vi "Initialize.vi"(6 "optional":variant, 8 "error in":errorcluster, 11 "FPGADMAChannelData in":refnum<class "FPGADMAChannelData.lvclass">) -> (0 "error out":errorcluster, 3 "Node*":refnum<data-value>)   [LabVIEW 2013, in "FPGADMAChannelData.lvclass"]
uses:
  FPGADMAChannelData.lvclass
  xCE/xceNode/xceNode.lvclass
  Categories/Categories.lvclass
  DMA_Read/DMA_Read.lvclass
  DMA_Write/DMA_Write.lvclass
  Category/Category.lvclass
  xCE/xceRootNode/xceRootNode.lvclass
  xCE/xceDataNode/xceDataNode.lvclass
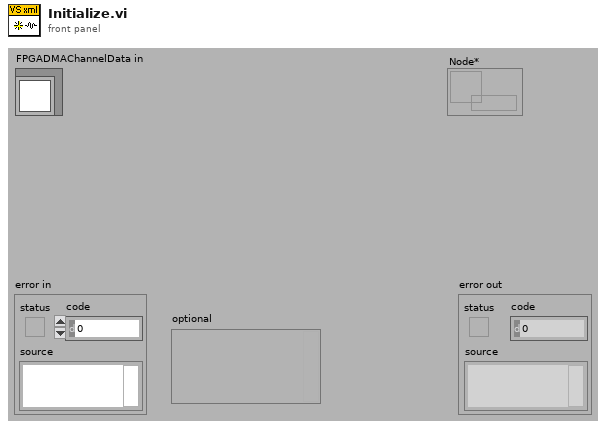
[diagram p1: front panel]
types:
  T1 = cluster{"className":string, "classAlias":string}[]
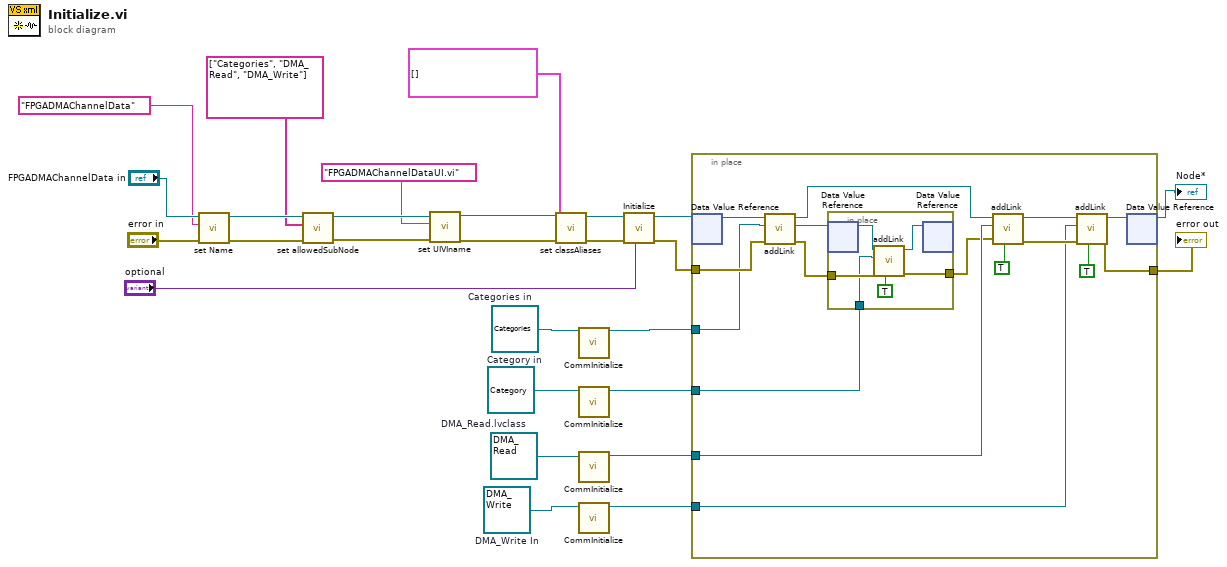
[diagram p0: block diagram]
diagram:
  w7 = refnum<class "Category.lvclass"> refnum  # Category in
  w13 = refnum<class "DMA_Write.lvclass"> refnum  # DMA_Write In
  w14 = refnum<class "DMA_Read.lvclass"> refnum  # DMA_Read.lvclass
  w15 = refnum<class "Categories.lvclass"> refnum  # Categories in
  n1 = call "set Name.vi"("error in (no error)"="error in", "Name"="FPGADMAChannelData", "xceDataNode in"="FPGADMAChannelData in") -> ("error out"=w22:errorcluster, "xceDataNode out"=w23:refnum<class "FPGADMAChannelData.lvclass">)  [unwired: 7 in]
  n2 = call "set allowedSubNode.vi"("error in (no error)"=w22, "Allowed subNode[]"=string[] ["Categories", "DMA_Read", "DMA_Write"], "xceDataNode in"=w23) -> ("error out"=w19:errorcluster, "xceDataNode out"=w20:refnum<class "FPGADMAChannelData.lvclass">)  [unwired: 7 in]
  n3 = call "set UIVIname.vi"("error in (no error)"=w19, "UI VI name"="FPGADMAChannelDataUI.vi", "xceDataNode in"=w20) -> ("error out"=w2:errorcluster, "xceDataNode out"=w5:refnum<class "FPGADMAChannelData.lvclass">)  [unwired: 7 in]
  n4 = call "set classAliases.vi"("error in (no error)"=w2, "classAliases"=T1 [], "xceRootNode in"=w5) -> ("error out"=w3:errorcluster, "xceRootNode out"=w4:refnum<class "FPGADMAChannelData.lvclass">)  [unwired: 7 in]
  n5 = call "CommInitialize.vi"("Categories in"=w15) -> ("Node*"=w12:refnum<data-value>)  [unwired: 9 in, 1 out]
  n6 = call "CommInitialize.vi"("Category in"=w7) -> ("Node*"=w6:refnum<data-value>)  [unwired: 9 in, 1 out]
  n7 = call "CommInitialize.vi"("DMA_Read.lvclass"=w14) -> ("Node*"=w11:refnum<data-value>)  [unwired: 9 in, 1 out]
  n8 = call "CommInitialize.vi"("DMA_Write In"=w13) -> ("Node*"=w10:refnum<data-value>)  [unwired: 9 in, 1 out]
  n9 = call-parent "Initialize.vi"("optional"="optional", "error in"=w3, "xceRootNode in"=w4) -> ("error out"=w16:errorcluster, "Node*"=w17:refnum<data-value>)  [unwired: 7 in]
  n10 = in-place {
    in-place-border: w16 -> [w39]
    in-place-border: w12 -> [w38]
    in-place-border: w11 -> [w37]
    in-place-border: w10 -> [w35]
    in-place-border: [w33] -> w9
    in-place-border: w6 -> [w28]
    n11 = in-place-dvr #1(w17) -> (w41:refnum<class "xceNode.lvclass">)  [unwired: 1 out]
    n12 = call "addLink.vi"("error in (no error)"=w39, "subNode in"=w38, "superNode in"=w41) -> ("error out"=w30:errorcluster, "subNode out"=w32:refnum<data-value>, "superNode out"=w31:refnum<class "xceNode.lvclass">)  [unwired: 6 in]
    n13 = in-place {
      in-place-border: w30 -> [w49]
      in-place-border: [w47] -> w29
      in-place-border: w28 -> [w46]
      n14 = in-place-dvr #2(w32) -> (w48:refnum<class "xceNode.lvclass">)  [unwired: 1 out]
      n15 = call "addLink.vi"("Append to End"=TRUE, "error in (no error)"=w49, "subNode in"=w46, "superNode in"=w48) -> ("error out"=w47:errorcluster, "superNode out"=w44:refnum<class "xceNode.lvclass">)  [unwired: 5 in, 1 out]
      n16 = in-place-dvr #2(w44) -> ()  [unwired: 2 out]
    }
    n17 = call "addLink.vi"("Append to End"=TRUE, "error in (no error)"=w29, "subNode in"=w37, "superNode in"=w31) -> ("error out"=w43:errorcluster, "superNode out"=w42:refnum<class "xceNode.lvclass">)  [unwired: 5 in, 1 out]
    n18 = call "addLink.vi"("Append to End"=TRUE, "error in (no error)"=w43, "subNode in"=w35, "superNode in"=w42) -> ("error out"=w33:errorcluster, "superNode out"=w40:refnum<class "xceNode.lvclass">)  [unwired: 5 in, 1 out]
    n19 = in-place-dvr #1(w40) -> (→"Node*":refnum<data-value>)  [unwired: 1 out]
  }
  "error out" <- w9
